vi "Max_Min_Measurement_Graph.vi"(1 "Graph Reference":refnum<vi>[](array[refnum]), 2 "Measurement Graphs (in)":T1[](array[typedef]) {"Y-Axis Array" items=["Time", "LI1CH1", "LI1CH2", "LI2CH1", "LI2CH2", "LI3CH1", "LI3CH2", "Field", "Temp", "Temp 2", "Temp 3", "N_Level", "H_Level", "Heat_370", "Sorb_Heat", "Still_Heat", "Capacity", "Loss", "Magnet_Temperature", "Lam_Pressure", "Lam_NValve", "370-T1", "370-T2", "370-T3", "370-T4", "370-T5", "370-R1", "370-R2", "370-R3", "370-R4", "370-R5", "372-T1", "372-T2", "372-T3", "372-T4", "372-T5", "372-T6", "372-R1", "372-R2", "372-R3", "372-R4", "372-R5", "372-R6", "Nada", "K2440_Res", "K2440_Current", "VTI_Heater", "VTI_NValve", "LS340_Heater", "K6221_Amplitude", "K6221_Frequency", "Cond_Pressure", "Still_Pressure", "FP_Out_Pressure", "Dump_Pressure", "V1", "V2", "V4", "V5", "V9", "Forepump", "Compressor", "K6221_Offset", "BoxTemp", "By", "Bz", "Phi", "heater-recond (%)", "Dewar Pressure ", "JT-SP-Control", "350 T1", "350 T2", "350 T3", "350 T4", "350 R1", "350 R2", "350 R3", "350 R4", "Angle"]; "X-Axis" items=["Time", "LI1CH1", "LI1CH2", "LI2CH1", "LI2CH2", "LI3CH1", "LI3CH2", "Field", "Temp", "Temp 2", "Temp 3", "N_Level", "H_Level", "Heat_370", "Sorb_Heat", "Still_Heat", "Capacity", "Loss", "Magnet_Temperature", "Lam_Pressure", "Lam_NValve", "370-T1", "370-T2", "370-T3", "370-T4", "370-T5", "370-R1", "370-R2", "370-R3", "370-R4", "370-R5", "372-T1", "372-T2", "372-T3", "372-T4", "372-T5", "372-T6", "372-R1", "372-R2", "372-R3", "372-R4", "372-R5", "372-R6", "Nada", "K2440_Res", "K2440_Current", "VTI_Heater", "VTI_NValve", "LS340_Heater", "K6221_Amplitude", "K6221_Frequency", "Cond_Pressure", "Still_Pressure", "FP_Out_Pressure", "Dump_Pressure", "V1", "V2", "V4", "V5", "V9", "Forepump", "Compressor", "K6221_Offset", "BoxTemp", "By", "Bz", "Phi", "heater-recond (%)", "Dewar Pressure ", "JT-SP-Control", "350 T1", "350 T2", "350 T3", "350 T4", "350 R1", "350 R2", "350 R3", "350 R4", "Angle"]}) -> (0 "Measurement Graphs (out)":T1[](array[typedef]) {"Y-Axis Array" items=["Time", "LI1CH1", "LI1CH2", "LI2CH1", "LI2CH2", "LI3CH1", "LI3CH2", "Field", "Temp", "Temp 2", "Temp 3", "N_Level", "H_Level", "Heat_370", "Sorb_Heat", "Still_Heat", "Capacity", "Loss", "Magnet_Temperature", "Lam_Pressure", "Lam_NValve", "370-T1", "370-T2", "370-T3", "370-T4", "370-T5", "370-R1", "370-R2", "370-R3", "370-R4", "370-R5", "372-T1", "372-T2", "372-T3", "372-T4", "372-T5", "372-T6", "372-R1", "372-R2", "372-R3", "372-R4", "372-R5", "372-R6", "Nada", "K2440_Res", "K2440_Current", "VTI_Heater", "VTI_NValve", "LS340_Heater", "K6221_Amplitude", "K6221_Frequency", "Cond_Pressure", "Still_Pressure", "FP_Out_Pressure", "Dump_Pressure", "V1", "V2", "V4", "V5", "V9", "Forepump", "Compressor", "K6221_Offset", "BoxTemp", "By", "Bz", "Phi", "heater-recond (%)", "Dewar Pressure ", "JT-SP-Control", "350 T1", "350 T2", "350 T3", "350 T4", "350 R1", "350 R2", "350 R3", "350 R4", "Angle"]; "X-Axis" items=["Time", "LI1CH1", "LI1CH2", "LI2CH1", "LI2CH2", "LI3CH1", "LI3CH2", "Field", "Temp", "Temp 2", "Temp 3", "N_Level", "H_Level", "Heat_370", "Sorb_Heat", "Still_Heat", "Capacity", "Loss", "Magnet_Temperature", "Lam_Pressure", "Lam_NValve", "370-T1", "370-T2", "370-T3", "370-T4", "370-T5", "370-R1", "370-R2", "370-R3", "370-R4", "370-R5", "372-T1", "372-T2", "372-T3", "372-T4", "372-T5", "372-T6", "372-R1", "372-R2", "372-R3", "372-R4", "372-R5", "372-R6", "Nada", "K2440_Res", "K2440_Current", "VTI_Heater", "VTI_NValve", "LS340_Heater", "K6221_Amplitude", "K6221_Frequency", "Cond_Pressure", "Still_Pressure", "FP_Out_Pressure", "Dump_Pressure", "V1", "V2", "V4", "V5", "V9", "Forepump", "Compressor", "K6221_Offset", "BoxTemp", "By", "Bz", "Phi", "heater-recond (%)", "Dewar Pressure ", "JT-SP-Control", "350 T1", "350 T2", "350 T3", "350 T4", "350 R1", "350 R2", "350 R3", "350 R4", "Angle"]})   [LabVIEW 2016]
uses:
  Monitor Communication/Plot.ctl
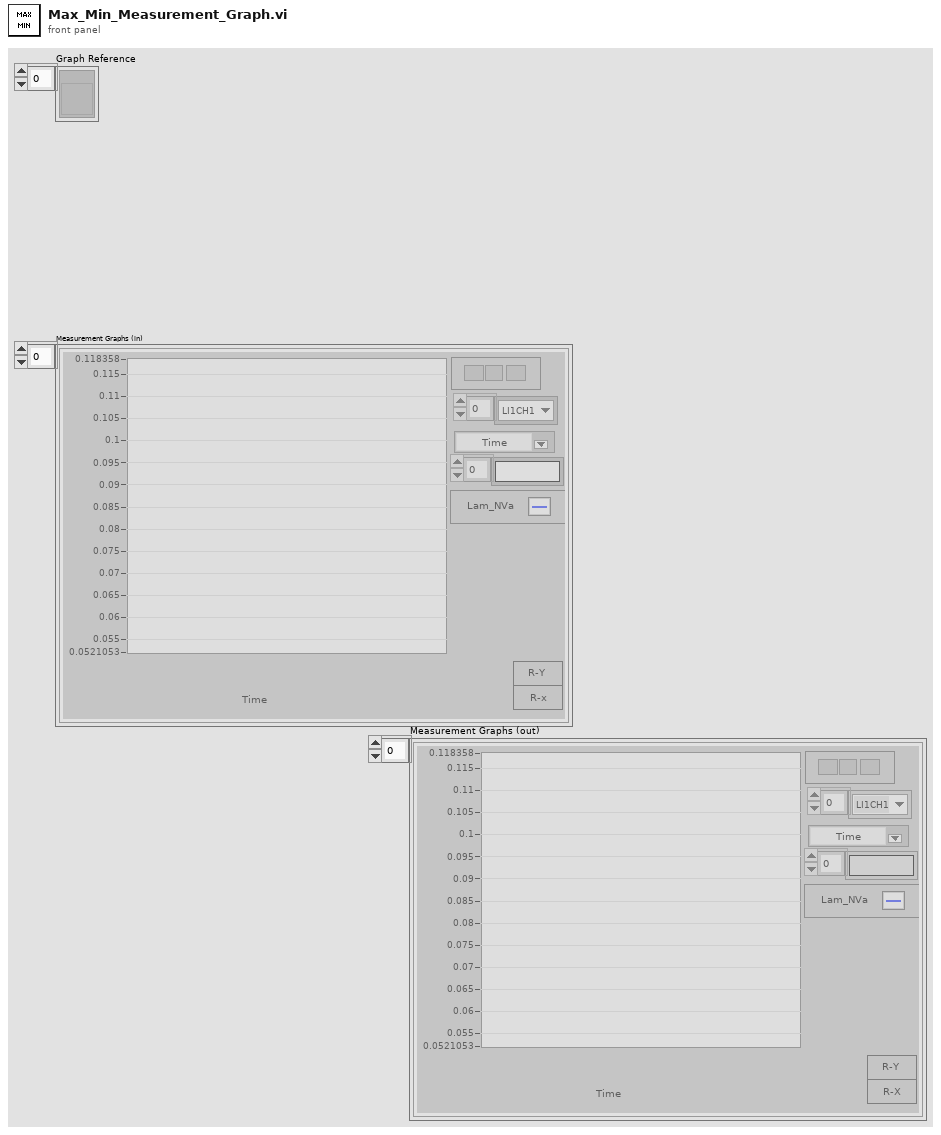
[diagram p1: front panel]
types:
  T1 = typedef "Plot.ctl" = cluster{"Measurement Graph":cluster{"Y":dbl[], "X":dbl[]}[], "X-Axis":i16, "Y-Axis Array":i16[], "Scale Plot":string[], "Rescale X":bool, "Rescale Y":bool}
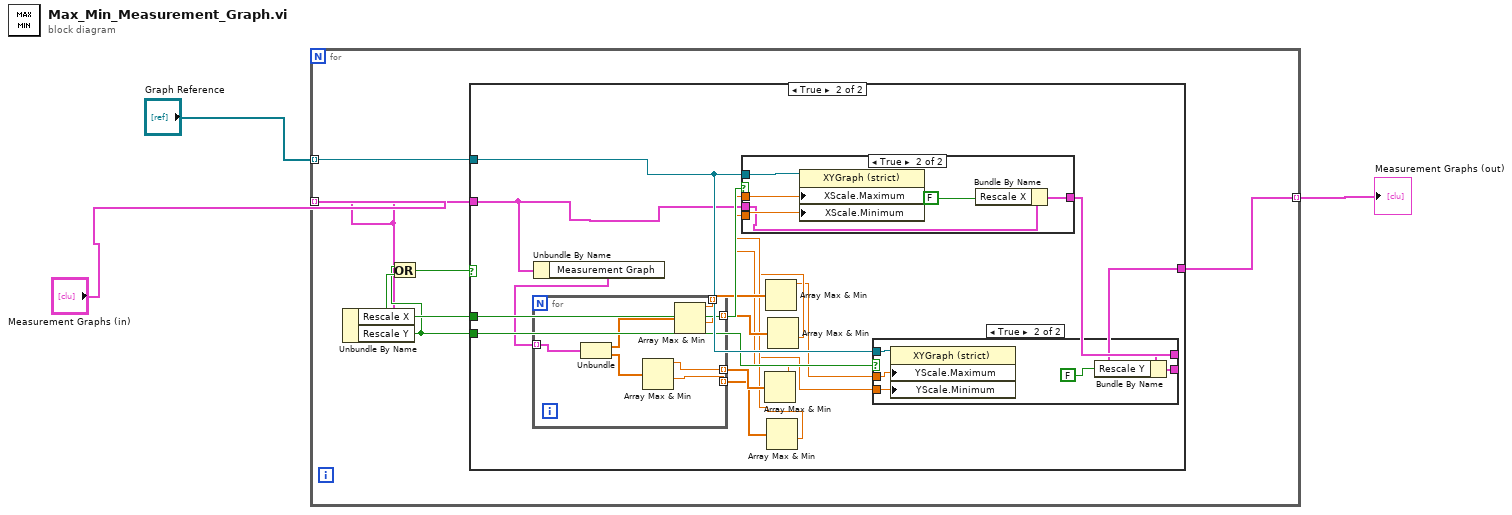
[diagram p0: block diagram]
diagram:
  n1 = for {
    tunnel: "Graph Reference" -> [w9] mode=indexing
    tunnel: "Measurement Graphs (in)" -> [w4] mode=indexing
    tunnel: [w8] -> w1 mode=indexing
    n2 = Unbundle By Name(w4) -> ("Rescale X"=w6:bool, "Rescale Y"=w5:bool)
    n3 = Or(x=w5, y=w6) -> (x .or. y?=w7:bool)
    n4 = case shown="True" w7 {
      tunnel: w9 -> [_ w23]
      tunnel: w4 -> [w10 w20]
      tunnel: [w10 w24] -> w8
      tunnel: w6 -> [_ w22]
      tunnel: w5 -> [_ w21]
      frame False {
      }
      frame True {
        n5 = Unbundle By Name(w20) -> ("Measurement Graph"=w11:cluster{"Y":dbl[], "X":dbl[]}[])
        n6 = for {
          tunnel: w11 -> [w30] mode=indexing
          tunnel: [w29] -> w19 mode=indexing
          tunnel: [w28] -> w18 mode=indexing
          tunnel: [w27] -> w17 mode=indexing
          tunnel: [w26] -> w16 mode=indexing
          n7 = Unbundle(w30) -> ("Y"=w32:dbl[], "X"=w31:dbl[])
          n8 = Array Max & Min(array=w31) -> (max value=w27:dbl, min value=w26:dbl)  [unwired: 2 out]
          n9 = Array Max & Min(array=w32) -> (max value=w29:dbl, min value=w28:dbl)  [unwired: 2 out]
        }
        n10 = Array Max & Min(array=w17) -> (max value=w15:dbl)  [unwired: 3 out]
        n11 = Array Max & Min(array=w19) -> (max value=w12:dbl)  [unwired: 3 out]
        n12 = Array Max & Min(array=w16) -> (min value=w14:dbl)  [unwired: 3 out]
        n13 = case shown="True" w22 {
          tunnel: w23 -> [_ w46]
          tunnel: w15 -> [_ w45]
          tunnel: w14 -> [_ w44]
          tunnel: w20 -> [w40 w43]
          tunnel: [w40 w41] -> w25
          frame False {
          }
          frame True {
            n14 = property on="Property Node" class="XYGraph (strict)"(reference=w46, "XScale.Maximum"=w45, "XScale.Minimum"=w44) -> ()  [unwired: 1 in, 2 out]
            n15 = Bundle By Name(cluster=w43, "Rescale X"=FALSE) -> (w41:T1)
          }
        }
        n16 = Array Max & Min(array=w18) -> (min value=w13:dbl)  [unwired: 3 out]
        n17 = case shown="True" w21 {
          tunnel: w25 -> [w33 w39]
          tunnel: [w33 w38] -> w24
          tunnel: w13 -> [_ w36]
          tunnel: w23 -> [_ w35]
          tunnel: w12 -> [_ w34]
          frame False {
          }
          frame True {
            n18 = property on="Property Node" class="XYGraph (strict)"(reference=w35, "YScale.Maximum"=w34, "YScale.Minimum"=w36) -> ()  [unwired: 1 in, 2 out]
            n19 = Bundle By Name(cluster=w39, "Rescale Y"=FALSE) -> (w38:T1)
          }
        }
      }
    }
  }
  "Measurement Graphs (out)" <- w1
